vi "Strings.vi"() -> ()   [LabVIEW 2010]
panel:
  in  "String 9":string
  in  "String 8":string
  in  "String 7":string
  in  "String 6":string
  in  "String 5":string
  in  "String 4":string
  in  "String 3":string
  in  "String 2":string
  in  "String":string
  # "Strings"
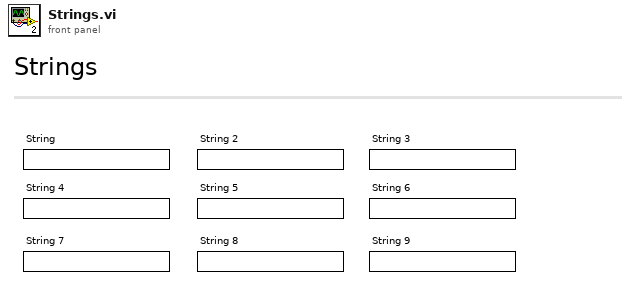
[diagram p1: front panel]
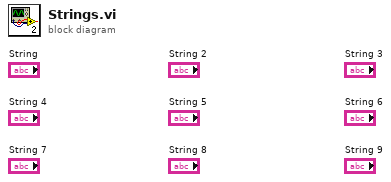
[diagram p0: block diagram]
diagram:
